vi "circularCounter32bitFxpStep.vi"(7 "reset":bool, 9 "doStep":bool=TRUE, 11 "maxCount":u32) -> (0 "maxReached":bool, 2 "next":u32, 3 "index":u32)   [LabVIEW 2015]
panel:
  in  "stepSize":fxp<+,16,2>
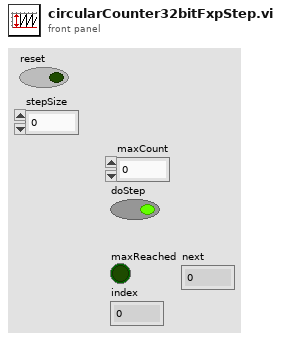
[diagram p1: front panel]
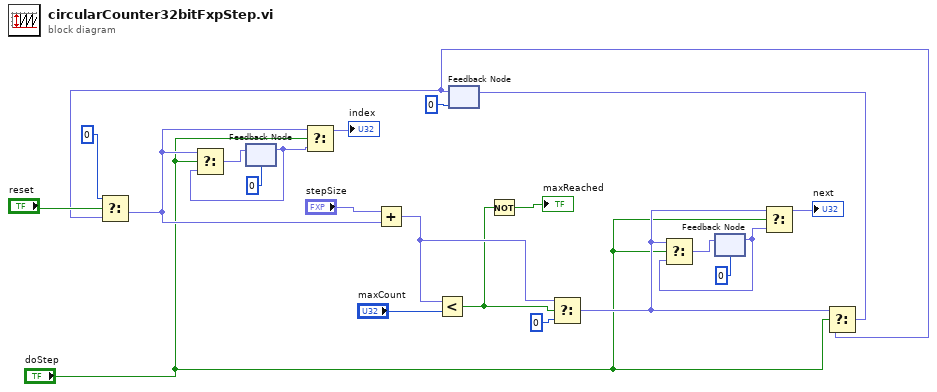
[diagram p0: block diagram]
diagram:
  n1 = feedback #1(u32 0) -> (w6:fxp<+/-,49,33>)
  n2 = feedback #2(u32 0) -> (w1:fxp<+/-,49,33>)
  n3 = Select(t=u32 0, s="reset", f=w1) -> (s? t:f=w5:fxp<+/-,49,33>)
  n4 = Select(t=w5, s="doStep", f=w6) -> (s? t:f=w7:fxp<+/-,49,33>)
  n5 = feedback-in #1(w7) -> ()
  n6 = Select(t=w5, s="doStep", f=w6) -> (s? t:f=→"index":fxp<+/-,49,33>)
  n7 = Add(x="stepSize", y=w5) -> (x+y=w20:fxp<+/-,32,16>)
  n8 = Less?(x=w20, y="maxCount") -> (x < y?=w18:bool)
  n9 = Not(x=w18) -> (.not. x?=→"maxReached":bool)
  n10 = Select(t=w20, s=w18, f=u32 0) -> (s? t:f=w11:fxp<+/-,49,33>)
  n11 = feedback #3(u32 0) -> (w9:fxp<+/-,49,33>)
  n12 = Select(t=w11, s="doStep", f=w9) -> (s? t:f=w12:fxp<+/-,49,33>)
  n13 = feedback-in #3(w12) -> ()
  n14 = Select(t=w11, s="doStep", f=w9) -> (s? t:f=→"next":fxp<+/-,49,33>)
  n15 = Select(t=w11, s="doStep", f=w1) -> (s? t:f=w17:fxp<+/-,49,33>)
  n16 = feedback-in #2(w17) -> ()
